vi "Write_Instr.vi"(8 "error in (no error)":errorcluster caption="entrée d'erreur (pas d'erreur)", 11 "Class Multimeter (Default) en entrée":refnum<class "Class Instrument Firebase Altyor.lvclass">) -> (0 "error out":errorcluster caption="sortie d'erreur", 3 "Class Multimeter (Default) en sortie":refnum<class "Class Instrument Firebase Altyor.lvclass">)   [LabVIEW 2020, in "Library Instrument & Equipement.lvlib" / "Library Instruments.lvlib" / "Class Instrument Firebase Altyor.lvclass"]
uses:
  Class Instrument Firebase Altyor.lvclass
  Class Instrument Firebase Altyor.lvclass/Class Instrument Firebase Altyor.ctl
  Instrument (Default)/Class Instrument (Default).lvclass
  Firebase/Source/Firebase Altyor/Firebase Altyor.lvclass
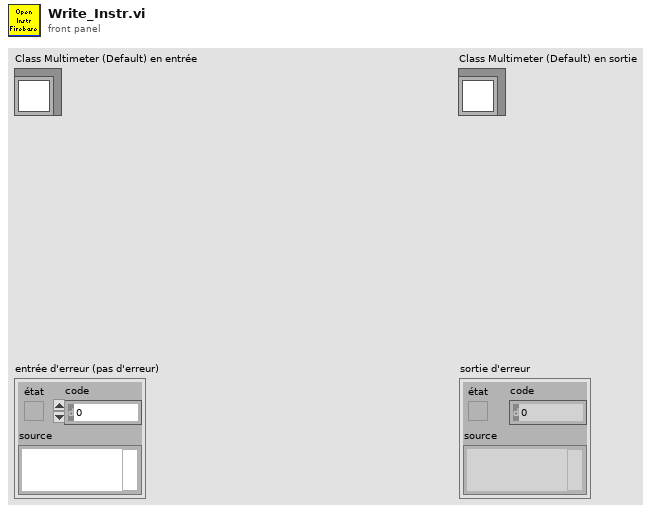
[diagram p1: front panel]
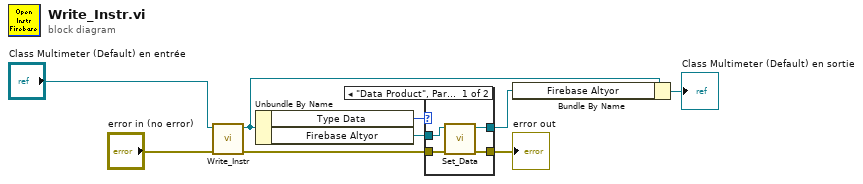
[diagram p0: block diagram]
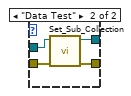
[diagram p2: hidden frame]
diagram:
  n1 = call-parent "Write_Instr.vi"("error in (no error)"="error in (no error)", "Class Multimeter (Default) en entrée"="Class Multimeter (Default) en entrée") -> ("error out"=w5:errorcluster, "Class Multimeter (Default) en sortie"=w3:refnum<class "Class Instrument Firebase Altyor.lvclass">)  [unwired: 8 in]
  n2 = Unbundle By Name(w3) -> ("Type Data"=w7:enum16{"Data Product", "Data Test"}, "Firebase Altyor"=w6:refnum<class "Firebase Altyor.lvclass">)
  n3 = case shown="\"Data Product\", Par défaut" w7 {
    tunnel: w5 -> [w11 w15]
    tunnel: [w13 w17] -> w4
    tunnel: w6 -> [w12 w16]
    tunnel: [w10 w14] -> w2
    frame "Data Product", Default {
      n4 = call-dynamic "Set_Data.vi"("error in (no error)"=w11, "Firebase Altyor en entrée"=w12) -> ("error out"=w13:errorcluster, "Firebase Altyor en sortie"=w10:refnum<class "Firebase Altyor.lvclass">)  [unwired: 8 in]
    }
    frame "Data Test" {
      n5 = call-dynamic "Set_Sub_Collection.vi"("error in (no error)"=w15, "Firebase PCBA en entrée"=w16) -> ("error out"=w17:errorcluster, "Firebase PCBA en sortie"=w14:refnum<class "Firebase Altyor.lvclass">)  [unwired: 8 in]
    }
  }
  "error out" <- w4
  n6 = Bundle By Name(cluster=w3, "Firebase Altyor"=w2) -> (→"Class Multimeter (Default) en sortie":refnum<class "Class Instrument Firebase Altyor.lvclass">)
